vi "Untitled 3 (SubVI) 1.vi"(6 "Array 3":dbl[](array[numeric]), 9 "Array in":dbl[](array[numeric]), 10 "Array 4":i32[](array[numeric]), 11 "Numeric":i32) -> (3 "Array out":dbl[](array[numeric]))   [LabVIEW 2013]
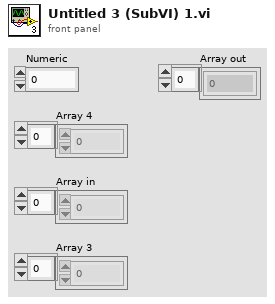
[diagram p1: front panel]
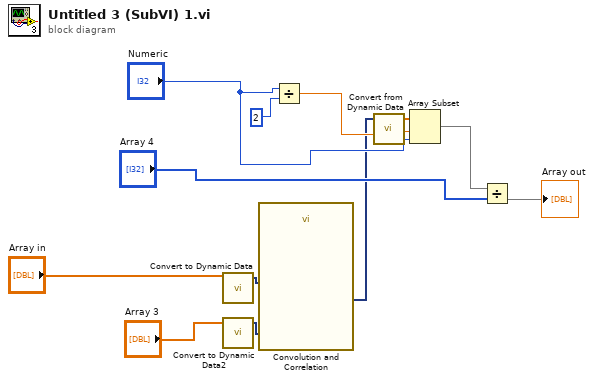
[diagram p0: block diagram]
diagram:
  n1 = call "Convert to Dynamic Data"("Array"="Array in") -> ("Dynamic Data Type"=w2:dynamicdata)  [unwired: 3 in]
  n2 = call "Convert to Dynamic Data2"("Array"="Array 3") -> ("Dynamic Data Type"=w9:dynamicdata)  [unwired: 3 in]
  n3 = call "Convolution and Correlation"("Y"=w9, "X"=w2) -> ("X*Y"=w3:dynamicdata)  [unwired: 8 in, 1 out]
  n4 = Divide(x="Numeric", y=2) -> (x/y=w7:dbl)
  n5 = call "Convert from Dynamic Data"("Dynamic Data Type"=w3) -> ("Array"=w4:dbl[])  [unwired: 3 in]
  n6 = Array Subset(array=w4, index=w7, length="Numeric") -> (w5:dbl[])
  n7 = Divide(x=w5, y="Array 4") -> (x/y=→"Array out":dbl[])
